vi "Create Plugin Interface Pool.vi"(7 "FIFO Debug Flags":refnum<class "FIFO Flags.lvclass">, 8 "error in (no error)":errorcluster, 11 "Plugin Interfaces":refnum<class "Plugin Interface.lvclass">[](array[class])) -> (0 "error out":errorcluster, 3 "Plugin Thread Pool out":refnum<class "Plugin Interface Pool.lvclass">)   [LabVIEW 2017, in "DSF Core.lvlib" / "Plugin Interface Pool.lvclass"]
uses:
  Plugin Interface Pool.lvclass
  C:/Git/DSF/Data Sharing Framework/Source/Core/Engine/Classes/Thread Pool/Pool.lvclass
  Interfaces/Transceiver Interface/Plugin Interface.lvclass
  C:/Git/DSF/Data Sharing Framework/Source/Core/Engine/Classes/Interfaces/Interface/Interface.lvclass
  Debug/FIFO Flags/FIFO Flags.lvclass
  Interfaces/Interface/Interface.lvclass/Interface.ctl
  Plugin Interface Pool.lvclass/Plugin Interface Pool.ctl
  Pool.lvclass
  Interfaces/Interface/Interface.lvclass
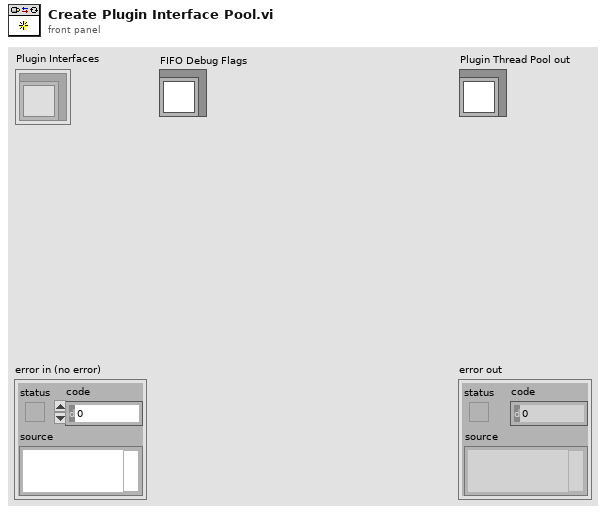
[diagram p1: front panel]
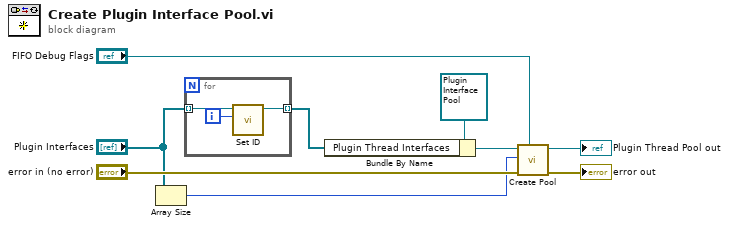
[diagram p0: block diagram]
diagram:
  n1 = Array Size(array="Plugin Interfaces") -> (size(s)=w4:i32)
  n2 = for {
    tunnel: "Plugin Interfaces" -> [w12] mode=indexing
    tunnel: [w10] -> w1 mode=indexing
    i -> [w11]
    n3 = call "Set ID.vi"("ID"=w11, "Interface in"=w12) -> ("Interface out"=w10:refnum<class "Plugin Interface.lvclass">)  [unwired: 9 in]
  }
  n4 = Bundle By Name(cluster=refnum<class "Plugin Interface Pool.lvclass"> refnum ("Plugin Thread Pool in"), "Plugin Thread Interfaces"=w1) -> (w7:refnum<class "Plugin Interface Pool.lvclass">)
  n5 = call "Create Pool.vi"("FIFO Debug Flags"="FIFO Debug Flags", "error in (no error)"="error in (no error)", "number of elements"=w4, "Pool type"=w7) -> ("error out"=→"error out":errorcluster, "Pool"=→"Plugin Thread Pool out":refnum<class "Plugin Interface Pool.lvclass">)  [unwired: 6 in]
